vi "Log Error.vi"(11 "Error In":errorcluster) -> (3 "Error Out":errorcluster)   [LabVIEW 2019]
uses:
  Log Level.ctl
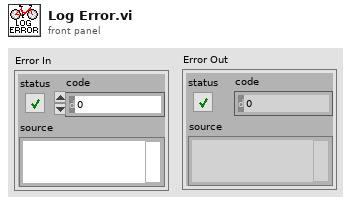
[diagram p1: front panel]
types:
  T1 = typedef "Log Level.ctl" = enum16{"Error", "Warning", "Info"}
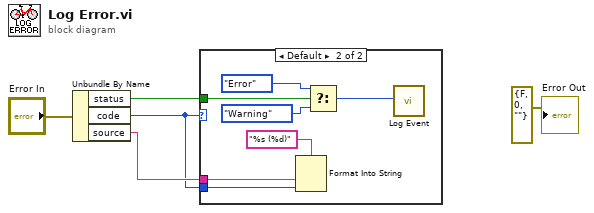
[diagram p0: block diagram]
diagram:
  n1 = Unbundle By Name("Error In") -> ("status"=w4:bool, "code"=w2:i32, "source"=w3:string)
  n2 = case shown="Default" w2 {
    tunnel: w4 -> [_ w12]
    tunnel: w3 -> [_ w7]
    tunnel: w2 -> [_ w6]
    frame 0 {
    }
    frame Default {
      n3 = Format Into String(format string="%s (%d)", w7, w6) -> ()  [unwired: 2 in, 2 out]
      n4 = Select(t=Log_Level."Error" ("Log Level"), s=w12, f=Log_Level."Warning" ("Log Level")) -> (s? t:f=w9:T1)
      n5 = call "Log Event.vi"("Log Level"=w9) -> ()  [unwired: 10 in, 1 out]
    }
  }
  "Error Out" <- errorcluster {"status"=FALSE, "code"=0, "source"=""} ("Error Out")
